vi "Search For Match.vi"(11 "Array":i32[](array[numeric])=[1, 1, 1, 1, 1, 1, 1, 1, 1, 1, 1, 1, 1, 1, 1, 1, 1, 1]) -> (2 "Index 2":i32, 3 "Index 1":i32)   [LabVIEW 2018]
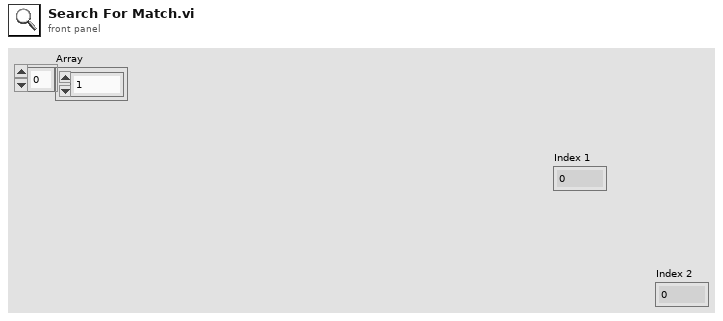
[diagram p1: front panel]
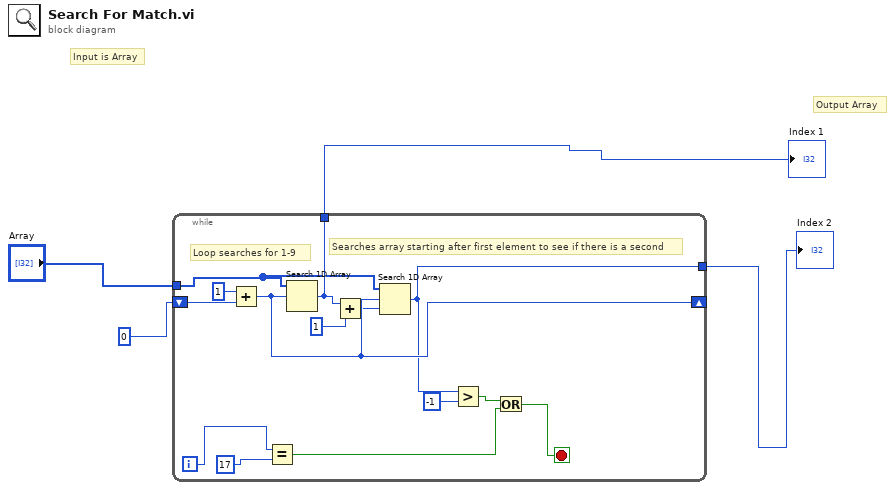
[diagram p0: block diagram]
diagram:
  # "Output Array"
  # "Input is Array"
  n1 = while {
    shift-right: [w16] -> _
    shift-left: 0 ("y") -> [w18]
    tunnel: [w12] -> w1
    tunnel: [w11] -> w2
    tunnel: "Array" -> [w6]
    i -> [w5]
    stop <- w7 stop-if-true
    # "Loop searches for 1-9"
    # "Searches array starting after first element to see if there is a second"
    n2 = Add(x=1, y=w18) -> (x+y=w16:i32)
    n3 = Equal?(x=w5, y=17) -> (x = y?=w8:bool)
    n4 = Search 1D Array(1D array=w6, element=w16) -> (index of element=w11:i32)  [unwired: 1 in]
    n5 = Add(x=w11, y=1) -> (x+y=w14:i32)
    n6 = Search 1D Array(1D array=w6, element=w16, start index (0)=w14) -> (index of element=w12:i32)
    n7 = Greater?(x=w12, y=-1) -> (0:w10:bool)
    n8 = Or(x=w10, y=w8) -> (x .or. y?=w7:bool)
  }
  "Index 1" <- w2
  "Index 2" <- w1
